vi "RefreshList.vi"(8 "error in (no error)":errorcluster, 11 "PLC_Module in":refnum<class "PLC_Module.lvclass">) -> (0 "error out":errorcluster, 3 "PLC_Module out":refnum<class "PLC_Module.lvclass">)   [LabVIEW 2025, in "PLC_Module.lvlib" / "PLC_Module.lvclass"]
uses:
  PLC_Module.lvclass
  PLC_Module.lvclass/PLC_Module.ctl
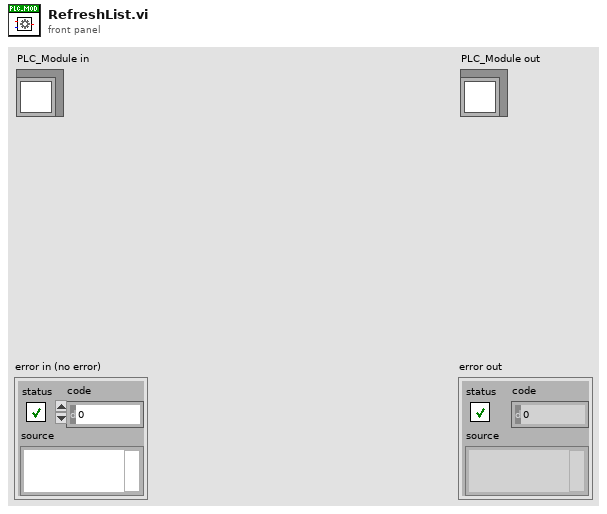
[diagram p1: front panel]
types:
  T1 = typedef "PLC_Module.lvlib/PLC_Module.lvclass/PLC_Data_Config.ctl" = map{string, cluster{"Config":T2, "Value":string}}
  T2 = typedef "PLC_Module.lvlib/PLC_Module.lvclass/PLC_Data.ctl" = cluster{"StartAddress":u32, "Direction":enum16{"PC->PLC", "PLC->PC"}, "DataType":T3, "DefaultValue":string, "Description":string}
  T3 = typedef "PLC_Module.lvlib/PLC_Module.lvclass/PLC_Data_Type.ctl" = enum16{"U8", "U32", "U32_Array", "String"}
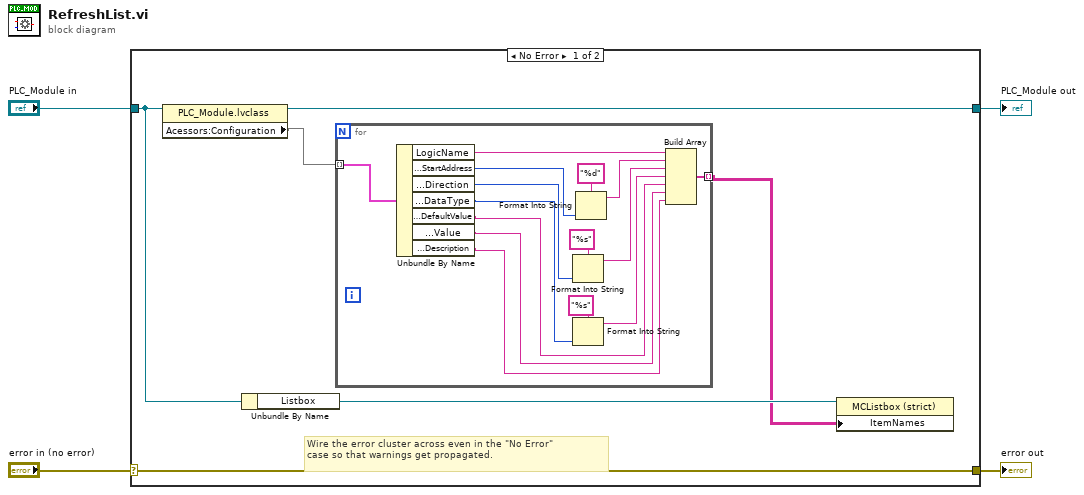
[diagram p0: block diagram]
diagram:
  n1 = case shown="No Error" "error in (no error)" {
    selector: "error in (no error)" -> [w10 w27]
    tunnel: [w10 w27] -> w3
    tunnel: [w9 w26] -> w1
    tunnel: "PLC_Module in" -> [w8 w26]
    frame No Error {
      # "Wire the error cluster across even in the \"No Error\"\ncase so that warnings get propagated."
      n2 = property class="PLC_Module.lvclass"(reference=w8) -> (reference out=w9:refnum<class "PLC_Module.lvclass">, "Acessors:Configuration"=w7:T1)  [unwired: 1 in, 1 out]
      n3 = Unbundle By Name(w8) -> ("Listbox"=w6:refnum<vi>)
      n4 = for {
        tunnel: w7 -> [w25] mode=indexing
        tunnel: [w11] -> w5 mode=indexing
        n5 = Unbundle By Name(w25) -> ("LogicName"=w23:string, "Config&Value.Config.StartAddress"=w24:u32, "Config&Value.Config.Direction"=w20:enum16{"PC->PLC", "PLC->PC"}, "Config&Value.Config.DataType"=w17:T3, "Config&Value.Config.DefaultValue"=w14:string, "Config&Value.Value"=w13:string, "Config&Value.Config.Description"=w12:string)
        n6 = Format Into String(format string="%s", w20) -> (resulting string=w18:string)  [unwired: 2 in, 1 out]
        n7 = Format Into String(format string="%s", w17) -> (resulting string=w15:string)  [unwired: 2 in, 1 out]
        n8 = Format Into String(format string="%d", w24) -> (resulting string=w22:string)  [unwired: 2 in, 1 out]
        n9 = Build Array(w23, w22, w18, w15, w14, w13, w12) -> (w11:string[])
      }
      n10 = property class="MCListbox (strict)"(reference=w6, "ItemNames"=w5) -> ()  [unwired: 1 in, 2 out]
    }
    frame Error {
    }
  }
  "error out" <- w3
  "PLC_Module out" <- w1
